vi "Estrazione fondo Host RT Test.vi"() -> ()   [LabVIEW 2014]
uses:
  <vilib>/FPGAPlugInAG/sbRIO-9636/niLvFpga_Open_sbRIO-9636.vi
  <vilib>/rvi/interface/common/dynamic/niFpgaDynamicAddResources.vi
  <vilib>/Utility/error.llb/Error Cluster From Error Code.vi
  <vilib>/rvi/errors/niLvFpgaAdjustHostInterfaceError.vi
  <vilib>/rvi/interface/common/niFpgaWaitOnOcc.vi
  <vilib>/FPGAPlugInAG/Dynamic/niLvFpga_Run_Dynamic.vi
  <vilib>/FPGAPlugInAG/Dynamic/niLvFpga_Reset_Dynamic.vi
  <vilib>/FPGAPlugInAG/Dynamic/niLvFpga_Abort_Dynamic.vi
  <vilib>/rvi/interface/nirviOpenFPGA/nirviOpenFPGA.xnode
  FPGA Bitfiles/LaserDistanceSen_FPGATarget_EstrazioneFondo-_j5tEHZ7DPrM.lvbitx
  FPGA Target/Support VIs/Estrazione Fondo - Target.vi
  <vilib>/rvi/interface/nirviReadWriteControl/nirviReadWriteControl.xnode
  <vilib>/rvi/interface/nirviMethod/nirviMethod.xnode
  <vilib>/FPGAPlugInAG/Dynamic/niLvFpga_ConfigureFifo_Dynamic.vi
  <vilib>/rvi/errors/niLvFpgaMergeErrorWithErrorCode.vi
  <vilib>/FPGAPlugInAG/Dynamic/niLvFpga_StartFifo_Dynamic.vi
  NiFpgaLv.dll
  <vilib>/rvi/interface/Simulation/niFpgaSimulationCallBeginRW.vi
panel:
  in  "polynomial order":i32=3
  in  "side points":i32=6
  out "Confronto Fondo-Segnale":dbl[][](graph)
  out "2^nbit misure":dbl
  out "Subtracted signal":dbl[](graph)
  in  "SubtractionType":T1(ring)
  out "Fondo Signal":dbl[](graph)
  out "Complete Mean Signal":dbl[](graph)
  in  "LowPass Filter: Low cutoff frequency":dbl=100000.0 format="%#_13g"
  in  "PolyFitting: Poly Grade":dbl=12.0
  in  "nbit":i32=8
  # "SavitzyGolay"
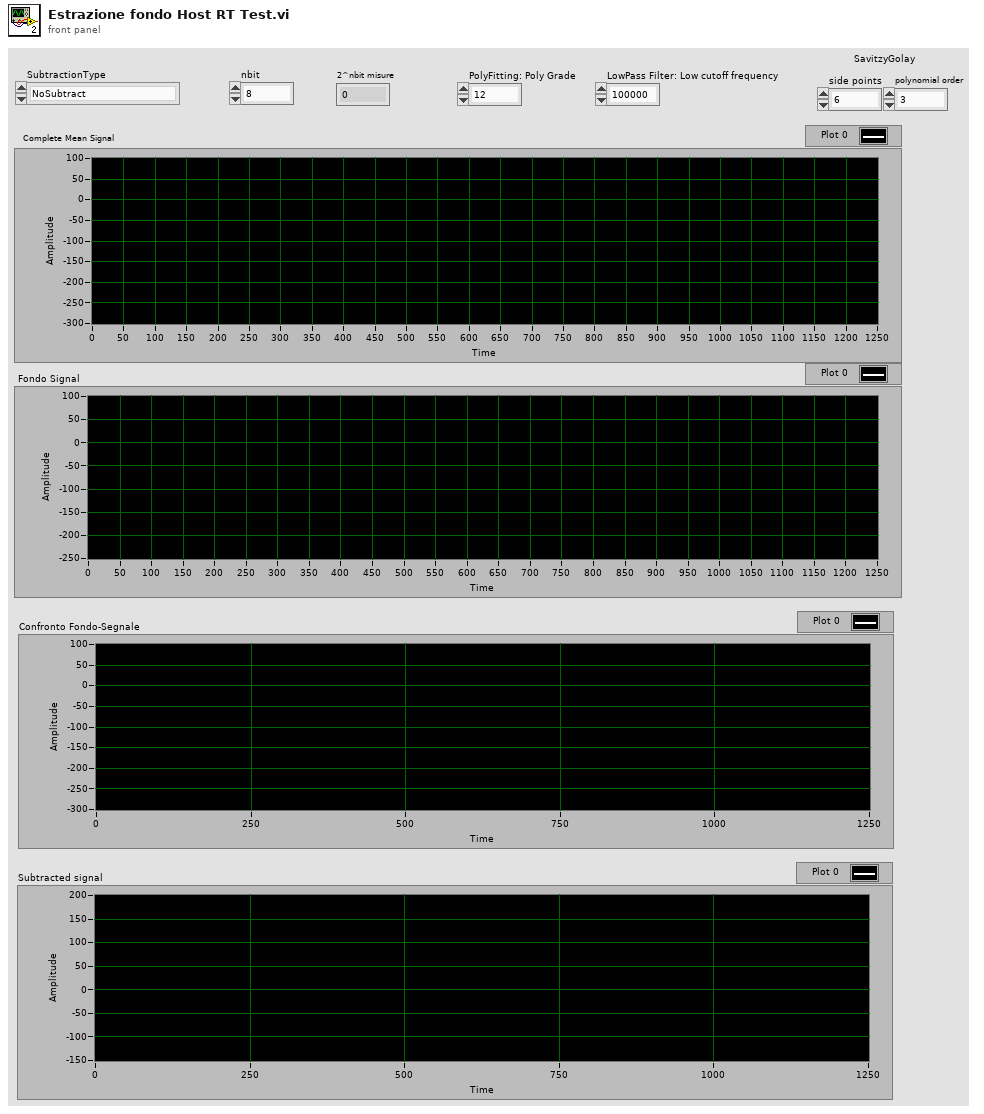
[diagram p1: front panel]
types:
  T1 = enum16{"NoSubtract", "StartingCurve", "LowPass", "PolyFitting", "SavGolay"}
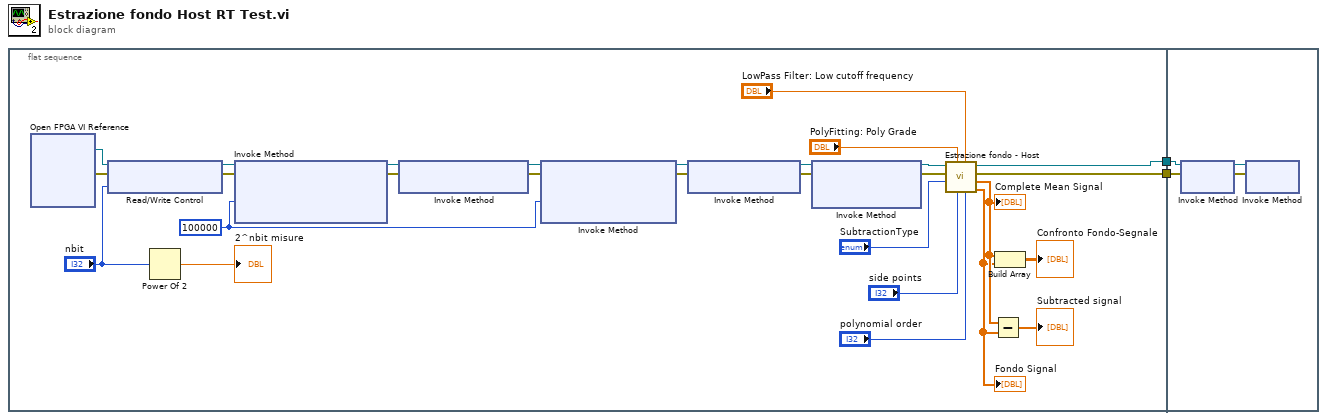
[diagram p0: block diagram]
diagram:
  n1 = flat-sequence {
    tunnel: [w16] -> w2
    tunnel: [w15] -> w1
    tunnel: w2 -> [w31]
    tunnel: w1 -> [w32]
    frame #0 {
      w28 = u32 100000 ("Requested Depth")
      n2 = xnode "Open FPGA VI Reference"() -> ("FPGA VI Reference Out"=w19:refnum<k20>, "error out"=w21:errorcluster)  [unwired: 2 in]
      n3 = xnode "Read/Write Control"("FPGA VI Reference In"=w19, "error in"=w21, "n-bit (2^nbit medie)"="nbit") -> ("FPGA VI Reference Out"=w18:refnum<k20>, "error out"=w20:errorcluster)
      n4 = Power Of 2(x="nbit") -> (2^x=→"2^nbit misure":dbl)
      n5 = xnode "Invoke Method"("FPGA VI Reference In"=w18, "error in"=w20, "Requested Depth"=w28) -> ("FPGA VI Reference Out"=w27:refnum<k20>, "error out"=w26:errorcluster)  [unwired: 1 out]
      n6 = xnode "Invoke Method"("FPGA VI Reference In"=w27, "error in"=w26) -> ("FPGA VI Reference Out"=w25:refnum<k20>, "error out"=w24:errorcluster)
      n7 = xnode "Invoke Method"("FPGA VI Reference In"=w25, "error in"=w24, "Requested Depth"=w28) -> ("FPGA VI Reference Out"=w30:refnum<k20>, "error out"=w29:errorcluster)  [unwired: 1 out]
      n8 = xnode "Invoke Method"("FPGA VI Reference In"=w30, "error in"=w29) -> ("FPGA VI Reference Out"=w23:refnum<k20>, "error out"=w22:errorcluster)
      n9 = xnode "Invoke Method"("FPGA VI Reference In"=w23, "error in"=w22) -> ("FPGA VI Reference Out"=w8:refnum<k20>, "error out"=w17:errorcluster)  [unwired: 1 in]
      n10 = call "Estrazione fondo - Host.vi"("polynomial order"="polynomial order", "LowPass Filter: Low cutoff frequency"="LowPass Filter: Low cutoff frequency", "side points"="side points", "PolyFitting: Poly Grade"="PolyFitting: Poly Grade", "SubtractionType"="SubtractionType", "error in"=w17, "FPGA VI Reference In"=w8) -> ("Fondo Signal"=w6:dbl[], "Complete Mean Signal"=w7:dbl[], "error out"=w16:errorcluster, "FPGA VI Reference Out"=w15:refnum<k20>)  [unwired: 1 in]
      "Complete Mean Signal" <- w7
      "Fondo Signal" <- w6
      n11 = Subtract(x=w7, y=w6) -> (x-y=→"Subtracted signal":dbl[])
      n12 = Build Array(w7, w6) -> (→"Confronto Fondo-Segnale":dbl[][])
    }
    frame #1 {
      n13 = xnode "Invoke Method"("FPGA VI Reference In"=w32, "error in"=w31) -> ("FPGA VI Reference Out"=w34:refnum<k20>, "error out"=w33:errorcluster)
      n14 = xnode "Invoke Method"("FPGA VI Reference In"=w34, "error in"=w33) -> ()  [unwired: 2 out]
    }
  }
